vi "IsMoving.vi"(8 "error in":errorcluster, 9 "Axis":enum16{"X", "Y", "Z"}(ring), 11 "VISA resource name":refnum<visa-resource-name>) -> (0 "error out":errorcluster, 2 "Is Ready?":bool, 3 "VISA resource name out":refnum<visa-resource-name>)   [LabVIEW 2017]
panel:
  out "element":u8 format="%x"
  out "Raw output (hex)":string
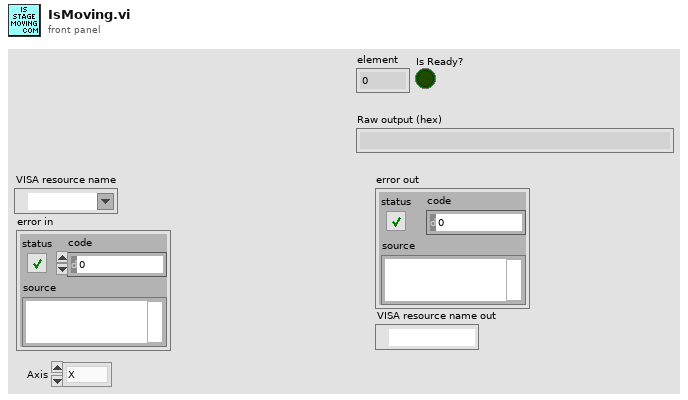
[diagram p1: front panel]
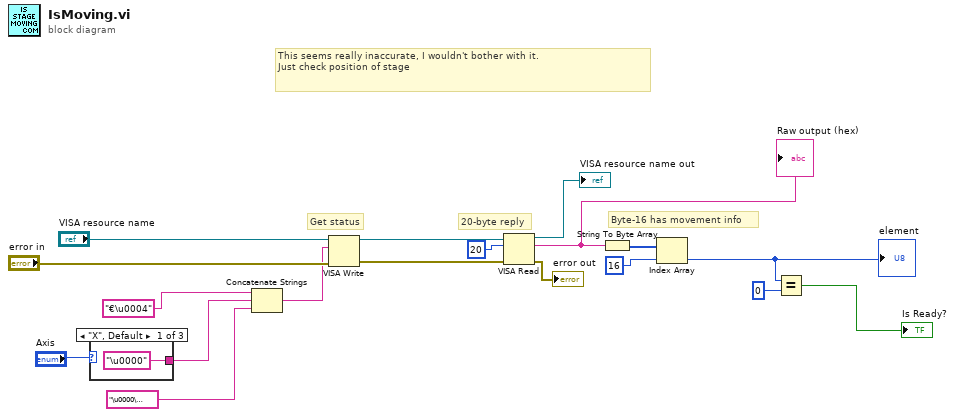
[diagram p0: block diagram]
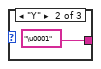
[diagram p2: hidden frame]
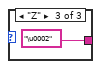
[diagram p3: hidden frame]
diagram:
  # "This seems really inaccurate, I wouldn't bother with it.\nJust check position of stage"
  # "20-byte reply"
  # "Get status"
  # "Byte-16 has movement info"
  n1 = case shown="\"X\", Default" "Axis" {
    tunnel: ["\u0000" "\u0001" "\u0002"] -> w14
    frame "X", Default {
    }
    frame "Y" {
    }
    frame "Z" {
    }
  }
  n2 = Concatenate Strings("€\u0004", w14, "\u0000\u0000\u0000") -> (w12:string)
  n3 = VISA Write(VISA resource name="VISA resource name", write buffer=w12, error in (no error)="error in") -> (VISA resource name out=w11:refnum<visa-resource-name>, error out=w9:errorcluster)  [unwired: 1 out]
  n4 = VISA Read(VISA resource name=w11, byte count=u32 20, error in (no error)=w9) -> (VISA resource name out=→"VISA resource name out":refnum<visa-resource-name>, read buffer=w8:string, error out=→"error out":errorcluster)  [unwired: 1 out]
  "Raw output (hex)" <- w8
  n5 = String To Byte Array(string=w8) -> (unsigned byte array=w7:u8[])
  n6 = Index Array(array=w7, index=16) -> (element=w3:u8)
  "element" <- w3
  n7 = Equal?(x=w3, y=u8 0) -> (x = y?=→"Is Ready?":bool)
